vi "To String.vi"(8 "error in (no error)":errorcluster, 11 "packed in":refnum<class "packed.lvclass">) -> (0 "error out":errorcluster, 2 "String":string, 3 "packed out":refnum<class "packed.lvclass">)   [LabVIEW 2020, in "Protobuf RAW.lvlib" / "packed.lvclass"]
uses:
  packed.lvclass
  packed.lvclass/packed.ctl
  Scalar Encoder/Scalar Type.lvclass
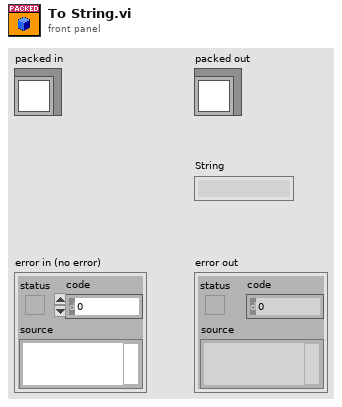
[diagram p1: front panel]
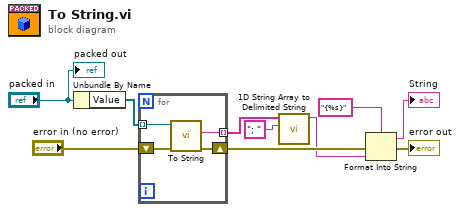
[diagram p0: block diagram]
diagram:
  n1 = Unbundle By Name("packed in") -> ("Value"=w6:refnum<class "Scalar Type.lvclass">[])
  n2 = for {
    tunnel: w6 -> [w14] mode=indexing
    shift-right: [w12] -> w5
    shift-left: "error in (no error)" -> [w13]
    tunnel: [w11] -> w4 mode=indexing
    n3 = call-dynamic "To String.vi"("error in (no error)"=w13, "Type Serializer in"=w14) -> ("error out"=w12:errorcluster, "String"=w11:string)  [unwired: 7 in, 1 out]
  }
  n4 = call <vilib>:"1D String Array to Delimited String.vi"("delimiter"="; ", "string array"=w4) -> ("delimited string"=w1:string)  [unwired: 9 in]
  n5 = Format Into String(format string="{%s}", error in=w5, w1) -> (resulting string=→"String":string, error out=→"error out":errorcluster)  [unwired: 1 in]
  "packed out" <- "packed in"
